vi "eliminate 999.vi"() -> ()   [LabVIEW 2012]
panel:
  out "Reported Turbidity":dbl
  out "all bad":bool
  out "sub data 2":T1(array[cluster])
  in  "failure rate":dbl=0.8
  out "number (0 to 1)":dbl
  out "x-1":i32
  out "elements":i32
  out "Previous data":T1(array[cluster])
  in  "ID":u16
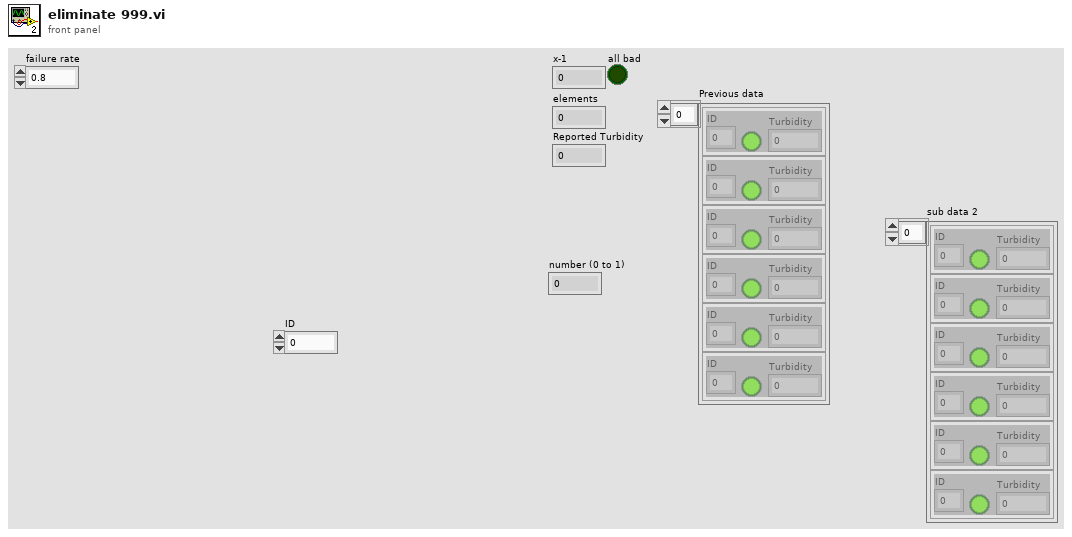
[diagram p1: front panel]
types:
  T1 = cluster{"ID":dbl, "Failed":bool, "Turbidity":dbl}[]
  T2 = cluster{"ID":dbl, "Failed":bool, "Turbidity":dbl}
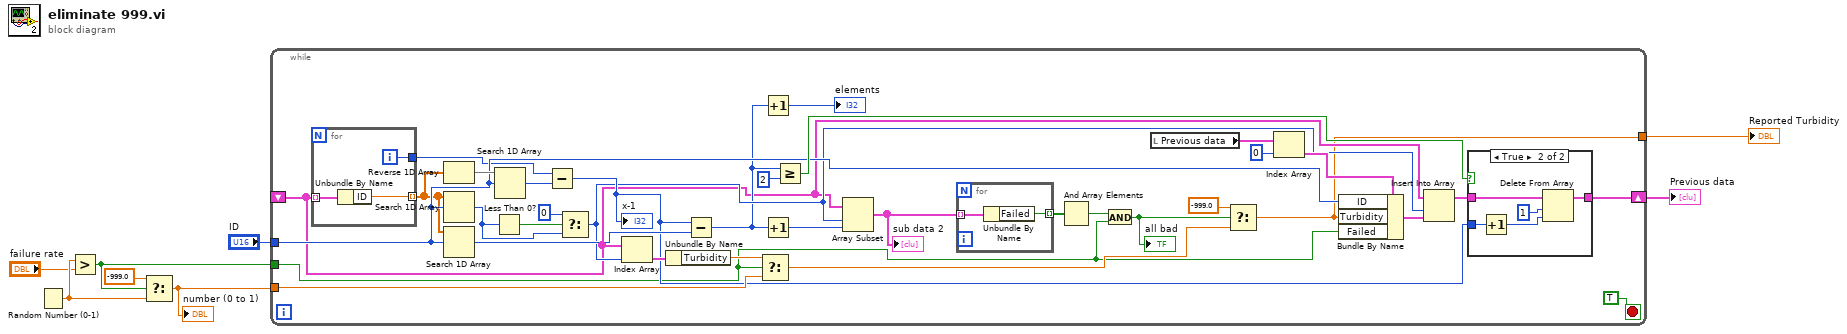
[diagram p0: block diagram]
diagram:
  n1 = Random Number (0-1)() -> (number: 0 to 1=w6:dbl)
  n2 = Greater?(x=w6, y="failure rate") -> (0:w5:bool)
  n3 = Select(t=-999.0, s=w5, f=w6) -> (s? t:f=w4:dbl)
  "number (0 to 1)" <- w4
  n4 = while {
    shift-right: [w34] -> w8
    shift-left: _ -> [w15]
    tunnel: w4 -> [w28]
    tunnel: w5 -> [w11]
    tunnel: "ID" -> [w29]
    tunnel: [w9] -> w1
    stop <- TRUE stop-if-true
    n5 = for {
      tunnel: w15 -> [w48] mode=indexing
      tunnel: [w47] -> w18 mode=indexing
      tunnel: [w46] -> w17
      i -> [w46]
      n6 = Unbundle By Name(w48) -> ("ID"=w47:dbl)
    }
    n7 = Reverse 1D Array(array=w18) -> (reversed array=w38:dbl[])
    n8 = Search 1D Array(1D array=w18, element=w29) -> (index of element=w31:i32)  [unwired: 1 in]
    n9 = Search 1D Array(1D array=w18, element=w29) -> (index of element=w33:i32)  [unwired: 1 in]
    n10 = Less Than 0?(x=w31) -> (x < 0?=w32:bool)
    n11 = Search 1D Array(1D array=w38, element=w29) -> (index of element=w37:i32)  [unwired: 1 in]
    n12 = Subtract(x=w17, y=w37) -> (x-y=w25:i32)
    "x-1" <- w25
    n13 = Select(t=0 ("index of element"), s=w32, f=w31) -> (s? t:f=w23:i32)
    n14 = Index Array(array=w15, index=w23) -> (element=w27:T2)
    n15 = Unbundle By Name(w27) -> ("Turbidity"=w26:dbl)
    n16 = Subtract(x=w25, y=w33) -> (x-y=w22:i32)
    n17 = Select(t=w26, s=w11, f=w28) -> (s? t:f=w13:dbl)
    n18 = Increment(x=w22) -> (x+1=→"elements":i32)
    n19 = Increment(x=w22) -> (x+1=w21:i32)
    n20 = Greater Or Equal?(x=w22, y=2) -> (x >= y?=w35:bool)
    n21 = Array Subset(array=w15, index=w23, length=w21) -> (w19:T1)
    "sub data 2" <- w19
    n22 = for {
      tunnel: w19 -> [w45] mode=indexing
      tunnel: [w44] -> w16 mode=indexing
      n23 = Unbundle By Name(w45) -> ("Failed"=w44:bool)
    }
    n24 = And Array Elements(Boolean array=w16) -> (logical AND=w12:bool)
    n25 = And(x=w12, y=w11) -> (x .and. y?=w10:bool)
    "all bad" <- w10
    n26 = local read "Previous data"() -> (w42:T1)
    n27 = Select(t=-999.0, s=w10, f=w13) -> (s? t:f=w9:dbl)
    n28 = Index Array(array=w42, index=0) -> (element=w40:T2)
    n29 = Bundle By Name(cluster=w40, "ID"=w29, "Turbidity"=w9, "Failed"=w11) -> (w39:T2)
    n30 = Insert Into Array(array=w15, index=w23, new element=w39) -> (w24:T1)
    n31 = case shown="True" w35 {
      tunnel: w24 -> [w49 w54]
      tunnel: [w49 w53] -> w34
      tunnel: w25 -> [_ w52]
      frame False {
      }
      frame True {
        n32 = Increment(x=w52) -> (x+1=w50:i32)
        n33 = Delete From Array(array=w54, length=1, index=w50) -> (array with subset deleted=w53:T1)  [unwired: 1 out]
      }
    }
  }
  "Previous data" <- w8
  "Reported Turbidity" <- w1
